vi "Get Configured Form Object.vi"(8 "error in (no error)":errorcluster, 10 "Table Name":string, 11 "Form from Configured Table in":refnum<class "Form from Configured Table.lvclass">) -> (0 "error out":errorcluster, 2 "Configured Form":refnum<class "Basic Form.lvclass">, 3 "Form from Configured Table out":refnum<class "Form from Configured Table.lvclass">)   [LabVIEW 2020, in "Panel Form Controller.lvlib" / "Form from Configured Table.lvclass"]
uses:
  Form from Configured Table.lvclass
  Database OOP/Table Libraries/Basic Form/Basic Form.lvclass
  Form from Configured Table.lvclass/Form from Configured Table.ctl
  Database OOP/Table Libraries/Table Configuration Interface/Table Configuration Interface.lvclass
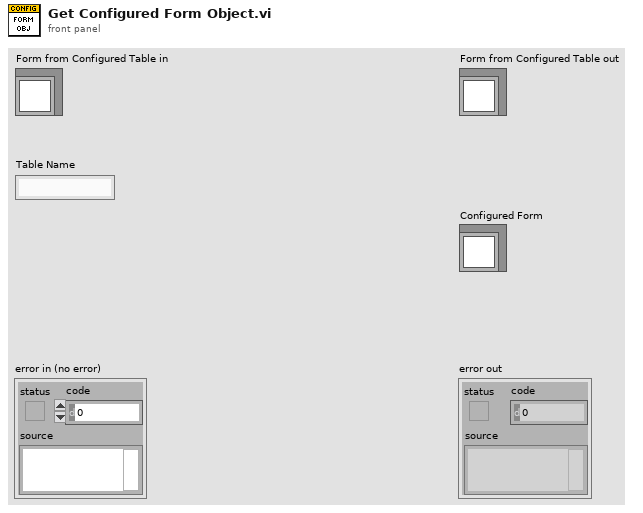
[diagram p1: front panel]
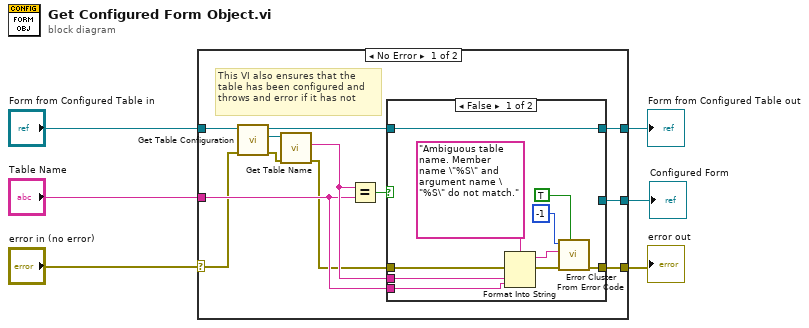
[diagram p0: block diagram]
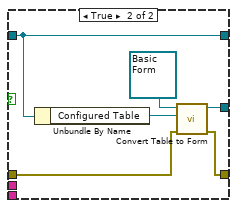
[diagram p2: hidden frame]
diagram:
  n1 = case shown="No Error" "error in (no error)" {
    selector: "error in (no error)" -> [w9 w36]
    tunnel: [w13 w36] -> w5
    tunnel: [w11 w35] -> w3
    tunnel: "Form from Configured Table in" -> [w18 w35]
    tunnel: "Table Name" -> [w14 _]
    tunnel: [w10 _] -> w1
    frame No Error {
      # "This VI also ensures that the table has been configured and\nthrows and error if it has not"
      n2 = call-dynamic "Get Table Configuration.vi"("error in (no error)"=w9, "Form from Configured Table in"=w18) -> ("error out"=w8:errorcluster, "Table Configuration"=w17:refnum<class "Table Configuration Interface.lvclass">, "Form from Configured Table out"=w12:refnum<class "Form from Configured Table.lvclass">)  [unwired: 7 in]
      n3 = call-dynamic "Get Table Name.vi"("error in (no error)"=w8, "Table Configuration Interface in"=w17) -> ("error out"=w7:errorcluster, "Table Name"=w15:string)  [unwired: 7 in, 1 out]
      n4 = Equal?(x=w15, y=w14) -> (x = y?=w16:bool)
      n5 = case shown="False" w16 {
        tunnel: w7 -> [w23 w30]
        tunnel: w15 -> [w22 _]
        tunnel: w14 -> [w21 _]
        tunnel: [w20 w29] -> w13
        tunnel: w12 -> [w19 w34]
        tunnel: [w19 w34] -> w11
        tunnel: [_ w31] -> w10
        frame False {
          n6 = Format Into String(format string="Ambiguous table name. Member name \"%S\" and argument name \"%S\" do not match.", error in=w23, w22, w21) -> (resulting string=w27:string, error out=w28:errorcluster)  [unwired: 1 in]
          n7 = call <vilib>:"Error Cluster From Error Code.vi"("show call chain? (False)"=TRUE, "error in (no error)"=w28, "error message (\"\")"=w27, "error code (0)"=-1) -> ("error out"=w20:errorcluster)  [unwired: 5 in]
        }
        frame True {
          n8 = Unbundle By Name(w34) -> ("Configured Table"=w33:refnum<class "Basic Table.lvclass">)
          n9 = call "Convert Table to Form.vi"("error in (no error)"=w30, "Table Object"=w33, "Basic Form in"=refnum<class "Basic Form.lvclass"> refnum ("Form.lvlib:Basic Form.lvclass")) -> ("error out"=w29:errorcluster, "Basic Form out"=w31:refnum<class "Basic Form.lvclass">)  [unwired: 7 in]
        }
      }
    }
    frame Error {
    }
  }
  "error out" <- w5
  "Form from Configured Table out" <- w3
  "Configured Form" <- w1
